vi "SaveTune.vi"(0 "Array":dbl[](array[numeric]), 1 "Save Data to File":bool, 2 "Ext time (sec)":dbl format="%#_10g", 3 "RawSignal":dbl[](array[numeric])) -> ()   [LabVIEW 2018]
uses:
  Global 2.vi
  MKS/Global - Pressure & Flow.vi
  RunNumberGlobal.vi
panel:
  out "Error Message":string
  out "Tune file name":string
  # "Save data to database"
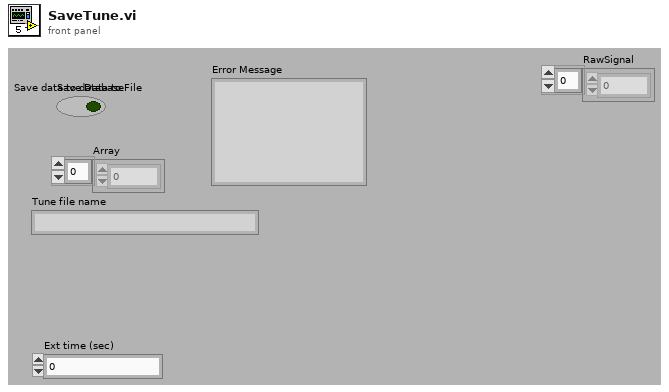
[diagram p1: front panel]
types:
  T1 = typedef "Control 1.ctl" = dbl
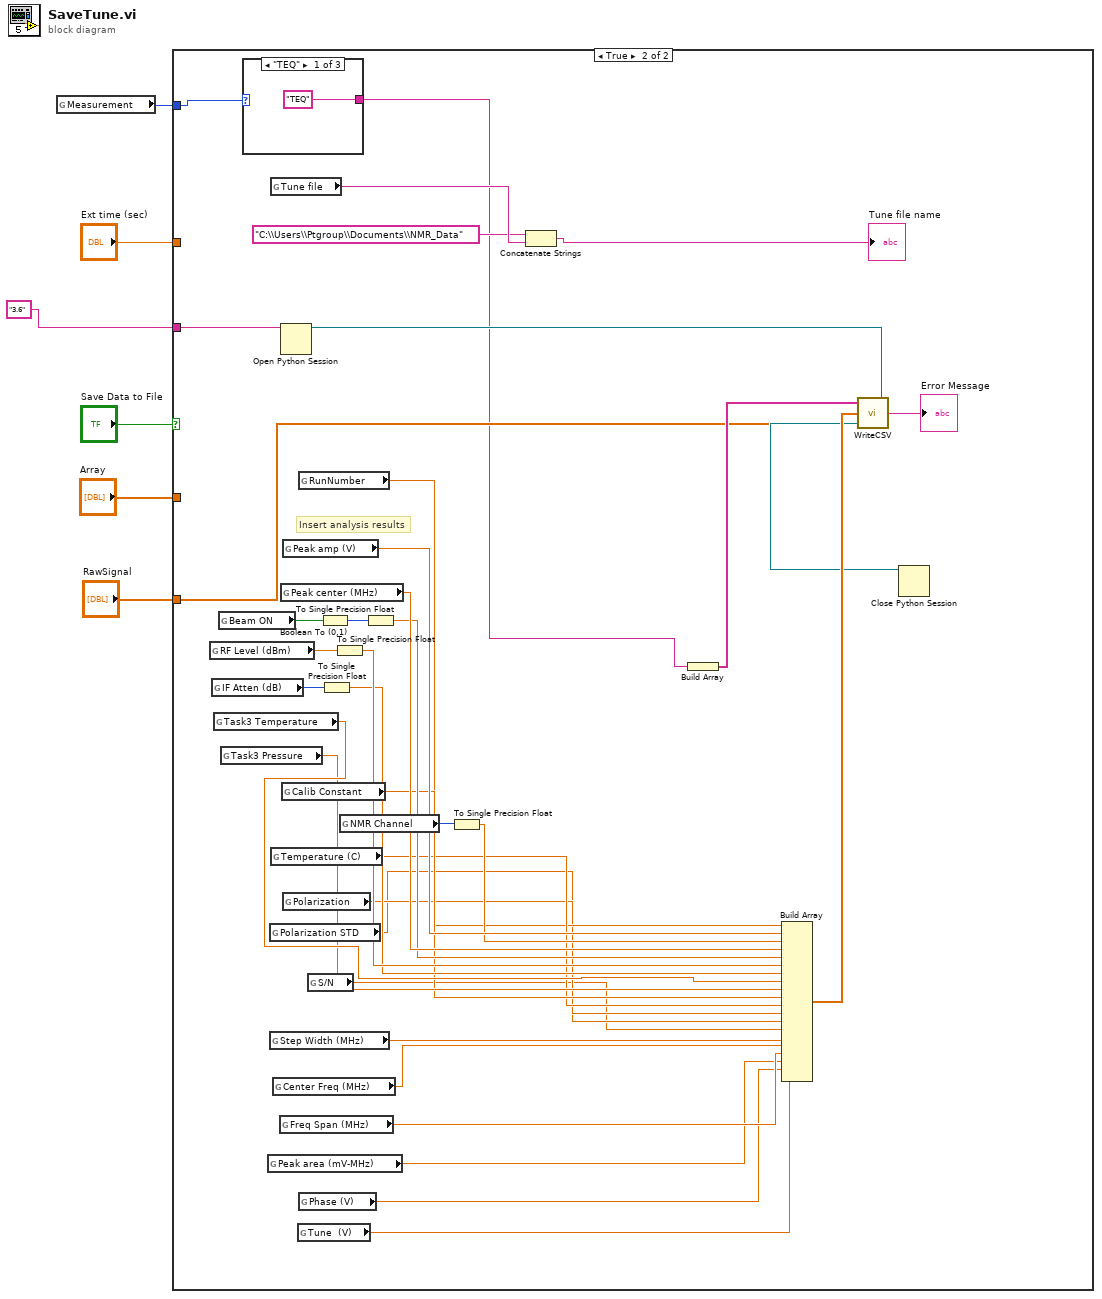
[diagram p0: block diagram]
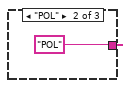
[diagram p3: hidden frame]
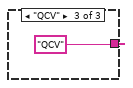
[diagram p4: hidden frame]
diagram:
  n1 = global read "Global 2.vi" "Measurement"() -> (w3:enum16{"TEQ", "POL", "QCV"})
  n2 = case shown="True" "Save Data to File" {
    tunnel: "Array" -> [_ _]
    tunnel: "Ext time (sec)" -> [_ _]
    tunnel: w3 -> [_ w20]
    tunnel: "3.6" ("Python version") -> [_ w26]
    tunnel: "RawSignal" -> [_ w21]
    frame False {
      # "Not writing file"
    }
    frame True {
      # "Insert analysis results"
      n3 = global read "Global 2.vi" "RF Level (dBm)"() -> (w36:dbl)
      n4 = global read "Global 2.vi" "IF Atten (dB)"() -> (w34:i8)
      n5 = global read "Global - Pressure & Flow.vi" "Task3 Temperature"() -> (w32:dbl)
      n6 = global read "Global 2.vi" "Beam ON"() -> (w38:bool)
      n7 = global read "Global - Pressure & Flow.vi" "Task3 Pressure"() -> (w31:dbl)
      n8 = case shown="\"TEQ\"" w20 {
        tunnel: ["TEQ" "POL" "QCV"] -> w7
        frame "TEQ" {
        }
        frame "POL" {
        }
        frame "QCV" {
        }
      }
      n9 = global read "Global 2.vi" "Peak area (mV-MHz)"() -> (w10:sgl)
      n10 = global read "Global 2.vi" "Polarization STD"() -> (w15:T1)
      n11 = global read "Global 2.vi" "Step Width (MHz)"() -> (w13:dbl)
      n12 = global read "Global 2.vi" "Tune file"() -> (w30:string)
      n13 = global read "Global 2.vi" "Temperature (C)"() -> (w18:dbl)
      n14 = global read "Global 2.vi" "Center Freq (MHz)"() -> (w12:dbl)
      n15 = global read "Global 2.vi" "Freq Span (MHz)"() -> (w11:dbl)
      n16 = Open Python Session(python version=w26) -> (session out=w25:refnum<k35>)  [unwired: 2 in, 1 out]
      n17 = global read "Global 2.vi" "Peak center (MHz)"() -> (w42:sgl)
      n18 = global read "Global 2.vi" "Calib Constant"() -> (w19:dbl)
      n19 = global read "Global 2.vi" "Peak amp (V)"() -> (w43:sgl)
      n20 = global read "Global 2.vi" "Polarization"() -> (w16:T1)
      n21 = global read "Global 2.vi" "Tune  (V)"() -> (w8:dbl)
      n22 = global read "RunNumberGlobal.vi" "RunNumber"() -> (w17:dbl)
      n23 = global read "Global 2.vi" "Phase (V)"() -> (w9:dbl)
      n24 = global read "Global 2.vi" "S/N"() -> (w14:dbl)
      n25 = Boolean To (0,1)(Boolean=w38) -> (0, 1=w39:i16)
      n26 = To Single Precision Float(number=w34) -> (single precision float=w33:sgl)
      n27 = To Single Precision Float(number=w36) -> (single precision float=w35:sgl)
      n28 = global read "Global 2.vi" "NMR Channel"() -> (w41:i32)
      n29 = To Single Precision Float(number=w39) -> (single precision float=w37:sgl)
      n30 = To Single Precision Float(number=w41) -> (single precision float=w40:sgl)
      n31 = Concatenate Strings("C:\\Users\\Ptgroup\\Documents\\NMR_Data", w30) -> (→"Tune file name":string)
      n32 = Build Array(w7) -> (w28:string[])
      n33 = Build Array(w17, w43, w40, w42, w37, w35, w33, w32, w31, w19, w18, w16, w15, w14, w13, w12, w11, w10, w9, w8) -> (w29:T1[])
      n34 = call "WriteCSV.vi"("session in"=w25, "Signal"=w21, "NumericData"=w29, "StringData"=w28) -> ("session out"=w24:refnum<k35>, "Error Message"=→"Error Message":string)
      n35 = Close Python Session(session in=w24) -> ()  [unwired: 1 in, 1 out]
    }
  }
